vi "cmd_set_loop_timer.vi"(8 "error in (no error)":errorcluster, 11 "JSON":string) -> (0 "error out":errorcluster)   [LabVIEW 2021]
doc: "Set interval of the FPGA main loop\n\n :param ticks: Specifies the interval in ticks"
uses:
  core/host_global_vars.vi
  <vilib>/Utility/error.llb/Error Cluster From Error Code.vi
  <vilib>/rvi/errors/niLvFpgaAdjustHostInterfaceError.vi
  <vilib>/rvi/interface/nirviReadWriteControl/nirviReadWriteControl.xnode
  FPGA Bitfiles/openlabspm_FPGATarget_fpgamain_eo-gUZR5D1g.lvbitx
  fpga/fpga_main.vi
  NiFpgaLv.dll
panel:
  in  "args":cluster{"val":u32}
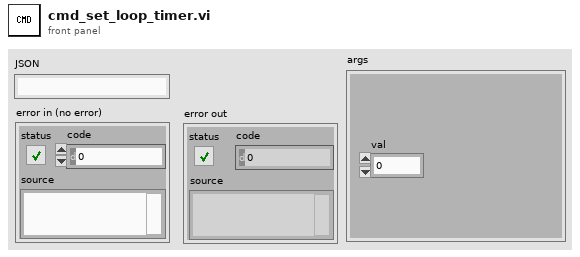
[diagram p1: front panel]
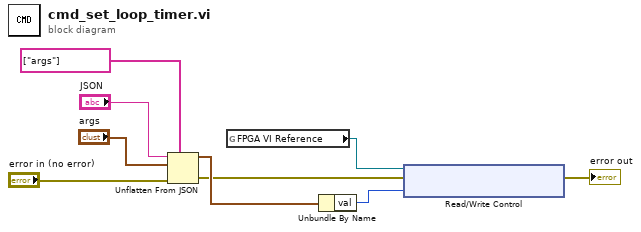
[diagram p0: block diagram]
diagram:
  n1 = Unflatten From JSON(path=string[] ["args"], JSON string="JSON", type and defaults="args", error in (no error)="error in (no error)") -> (value=w5:cluster{"val":u32}, error out=w2:errorcluster)  [unwired: 3 in]
  n2 = global read "host_global_vars.vi" "FPGA VI Reference"() -> (w3:refnum<k20>)
  n3 = Unbundle By Name(w5) -> ("val"=w1:u32)
  n4 = xnode "Read/Write Control"("FPGA VI Reference In"=w3, "error in"=w2, "loop timer"=w1) -> ("error out"=→"error out":errorcluster)  [unwired: 1 out]
